vi "Flow_signal_scaling.vi"(11 "data":waveform(dbl)[](array[waveform])) -> (3 "Array":waveform(dbl)[](array[waveform]))   [LabVIEW 2016]
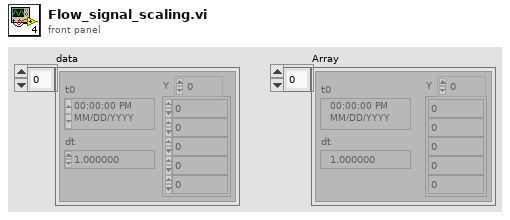
[diagram p1: front panel]
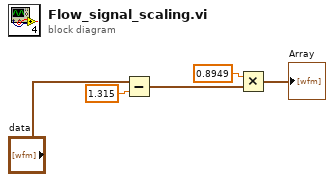
[diagram p0: block diagram]
diagram:
  n1 = Subtract(x="data", y=1.315) -> (x-y=w3:waveform(dbl)[])
  n2 = Multiply(x=0.8949, y=w3) -> (x*y=→"Array":waveform(dbl)[])
